vi "Demo1.vi"() -> ()   [LabVIEW 2020]
uses:
  <vilib>/Utility/file.llb/Read Delimited Spreadsheet (I64).vi
panel:
  out "indicator":bool
  in  "OK Button":bool
  out "new file path (Not A Path if cancelled)":path
  out "all rows":i64[][](array[numeric])
  out "number":i32
  out "Status":string
  out "Pass/Fail":bool
  in  "A 2":i32=5
  in  "B 2":i32=1
  out "Result 2":i32
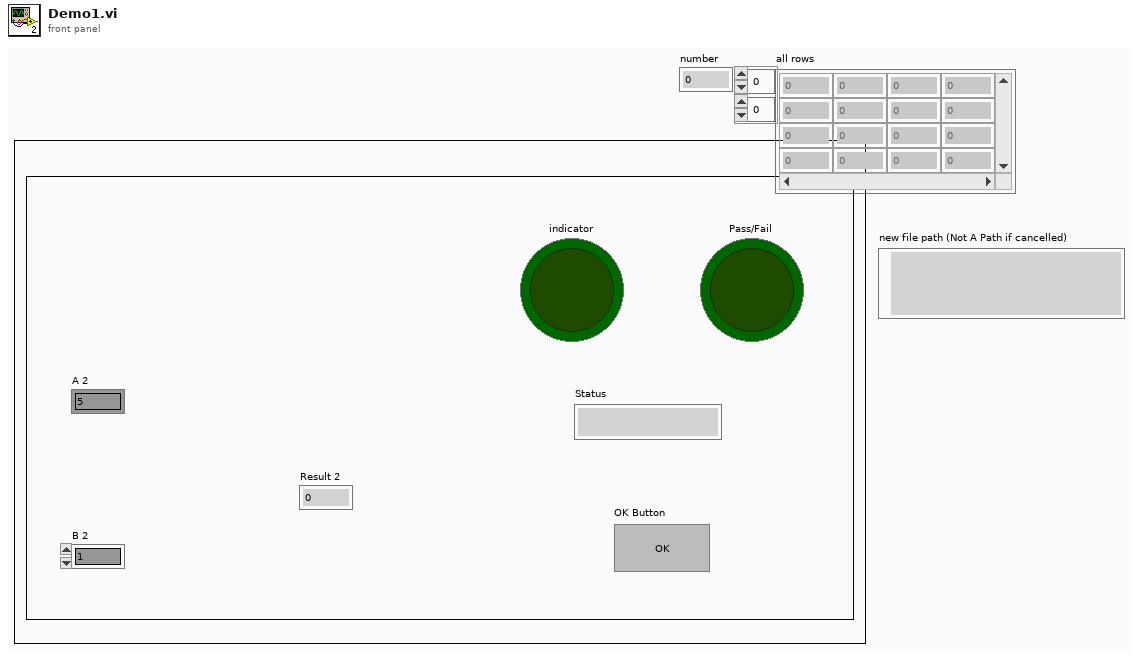
[diagram p1: front panel]
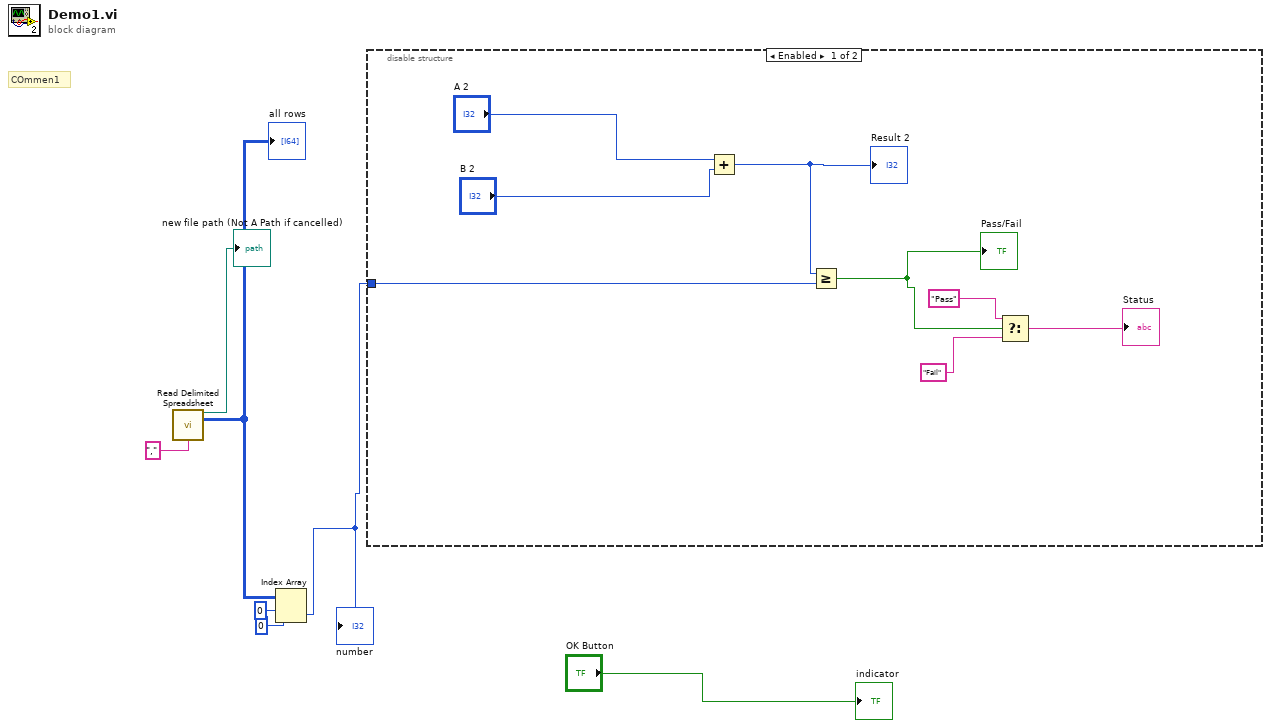
[diagram p0: block diagram]
diagram:
  # "COmmen1"
  n1 = call-poly <vilib>:"Read Delimited Spreadsheet.vi"("delimiter (\\t)"="," ("delimiter (\\t)")) -> ("new file path (Not A Path if cancelled)"=→"new file path (Not A Path if cancelled)":path, "all rows"=w7:i64[][])  [unwired: 9 in, 4 out]
  "all rows" <- w7
  n2 = Index Array(array=w7, index (row)=0, index (col)=0 ("disabled index (col)")) -> (element=w4:i64)
  "number" <- w4
  n3 = disable-structure shown="Enabled" {
    disable-tunnel: w4 -> [w8 _]
    frame Enabled {
      n4 = Add(x="A 2", y="B 2") -> (x+y=w13:i32)
      "Result 2" <- w13
      n5 = Greater Or Equal?(x=w13, y=w8) -> (x >= y?=w12:bool)
      "Pass/Fail" <- w12
      n6 = Select(t="Pass", s=w12, f="Fail") -> (s? t:f=→"Status":string)
    }
    frame Disabled {
    }
  }
  "indicator" <- "OK Button"
